vi "Update Panels.vi"(10 "Apps":refnum<class "ViaApp.lvclass">[](array[class]), 11 "PanelArray":refnum<class "ArrayManager.lvclass">) -> ()   [LabVIEW 2020, in "PicoG-App.lvlib" / "AppListPanel.lvclass"]
uses:
  AppListPanel.lvclass
  <vilib>/IlluminatedG/IG OOPanel/OOPanel/ArrayManager/ArrayManager.lvclass
  ViaApp/ViaApp.lvclass
  GWebAppArrayPanel/GWebAppArrayPanel.lvclass
  C:/Program Files (x86)/National Instruments/LabVIEW 2020/vi.lib/IlluminatedG/IG OOPanel/OOPanel/ArrayPanel/ArrayPanel.lvclass
  Sort By Updated.vi
  <vilib>/IlluminatedG/IG OOPanel/OOPanel/Panel/Panel.lvclass
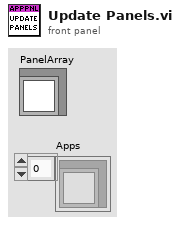
[diagram p1: front panel]
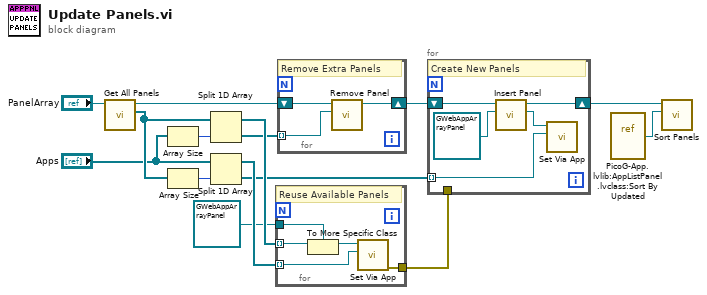
[diagram p0: block diagram]
diagram:
  n1 = call <vilib>:"Get All Panels.vi"("PanelArray in"="PanelArray") -> ("Panels"=w14:refnum<class "ArrayPanel.lvclass">[], "PanelArray out"=w8:refnum<class "ArrayManager.lvclass">)  [unwired: 8 in, 1 out]
  n2 = Array Size(array="Apps") -> (size(s)=w13:i32)
  n3 = Array Size(array=w14) -> (size(s)=w11:i32)
  n4 = Split 1D Array(array=w14, index=w13) -> (first subarray=w10:refnum<class "ArrayPanel.lvclass">[], second subarray=w7:refnum<class "ArrayPanel.lvclass">[])
  n5 = Split 1D Array(array="Apps", index=w11) -> (first subarray=w9:refnum<class "ViaApp.lvclass">[], second subarray=w5:refnum<class "ViaApp.lvclass">[])
  n6 = for {
    tunnel: w9 -> [w18] mode=indexing
    tunnel: w10 -> [w20] mode=indexing
    tunnel: [w17] -> w4
    tunnel: refnum<class "GWebAppArrayPanel.lvclass"> refnum ("PicoG-App.lvlib:GWebAppArrayPanel.lvclass") -> [w16]
    # "Reuse Available Panels"
    n7 = To More Specific Class(target class=w16, reference=w20) -> (specific class reference=w19:refnum<class "GWebAppArrayPanel.lvclass">)  [unwired: 1 in, 1 out]
    n8 = call "Set Via App.vi"("ViaApp"=w18, "GWebAppArrayPanel in"=w19) -> ("error out"=w17:errorcluster)  [unwired: 8 in, 1 out]
  }
  n9 = for {
    tunnel: w7 -> [w22] mode=indexing
    shift-right: [w21] -> w6
    shift-left: w8 -> [w23]
    # "Remove Extra Panels"
    n10 = call <vilib>:"Remove Panel.vi"("Panel in"=w22, "ArrayManager in"=w23) -> ("ArrayManager out"=w21:refnum<class "ArrayManager.lvclass">)  [unwired: 7 in, 2 out]
  }
  n11 = for {
    shift-right: [w27] -> w3
    shift-left: w6 -> [w28]
    tunnel: w5 -> [w24] mode=indexing
    tunnel: w4 -> [_]
    # "Create New Panels"
    n12 = call <vilib>:"Insert Panel.vi"("Panel/Type"=refnum<class "GWebAppArrayPanel.lvclass"> refnum ("PicoG-App.lvlib:GWebAppArrayPanel.lvclass"), "PanelArray in"=w28) -> ("Panel"=w25:refnum<class "GWebAppArrayPanel.lvclass">, "PanelArray out"=w27:refnum<class "ArrayManager.lvclass">)  [unwired: 7 in, 1 out]
    n13 = call "Set Via App.vi"("ViaApp"=w24, "GWebAppArrayPanel in"=w25) -> ()  [unwired: 8 in, 2 out]
  }
  n14 = vi-ref "PicoG-App.lvlib:AppListPanel.lvclass:Sort By Updated.vi"() -> (w2:refnum<vi>)
  n15 = call <vilib>:"Sort Panels.vi"("Sort VI"=w2, "ArrayManager in"=w3) -> ()  [unwired: 8 in, 2 out]
